vi "Test SyncStart 2.vi"() -> ()   [LabVIEW 2017]
uses:
  274801fc-fe2a-4412-a660-e416e3d3dfa2.vi
  e6d22657-482a-40f8-b9e6-8851e5ea81f9.vi
  9ccd6827-3ff4-4c10-ac1b-fb27d356ceb2.vi
  815a932d-7b12-48c6-9f28-7d788b7c90a6.vi
  25f0e5d1-a262-4e62-8561-2edca888c82f.vi
  Synchronization/SyncStart/_Obtain SyncStart Queue.vi
panel:
  in  "state 3":bool
  in  "state 2":bool
  in  "state 1":bool
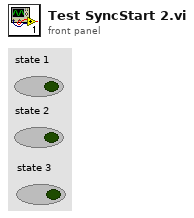
[diagram p1: front panel]
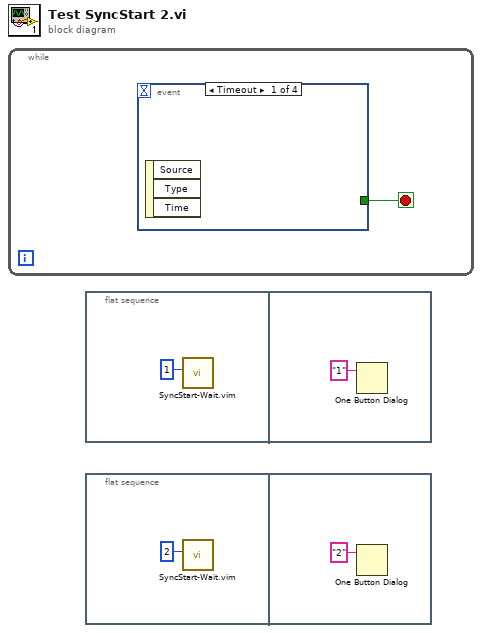
[diagram p0: block diagram]
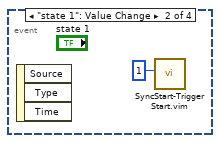
[diagram p2: hidden frame]
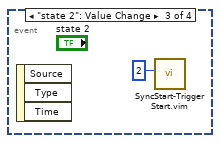
[diagram p3: hidden frame]
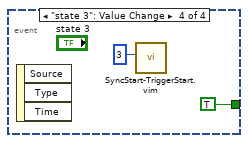
[diagram p4: hidden frame]
diagram:
  n1 = while {
    stop <- w1 stop-if-true
    n2 = event shown="[0] Timeout" {
      selector: _ -> [_ _ _ _]
      dyn-events: _ -> [_ _ _ _]
      timeout: _ -> [_ _ _ _]
      tunnel: [_ _ _ TRUE] -> w1
      event Timeout {
        n3 = event-data() -> ()  [unwired: 1 in, 3 out]
      }
      event "state 1": Value Change {
        n4 = event-data() -> ()  [unwired: 1 in, 3 out]
        n5 = call "SyncStart-TriggerStart.vim"("state(Enum or Int)"=1 ("state")) -> ()  [unwired: 10 in, 1 out]
      }
      event "state 2": Value Change {
        n6 = event-data() -> ()  [unwired: 1 in, 3 out]
        n7 = call "SyncStart-TriggerStart.vim"("state(Enum or Int)"=2 ("state")) -> ()  [unwired: 10 in, 1 out]
      }
      event "state 3": Value Change {
        n8 = event-data() -> ()  [unwired: 1 in, 3 out]
        n9 = call "SyncStart-TriggerStart.vim"("state(Enum or Int)"=3 ("state")) -> ()  [unwired: 10 in, 1 out]
      }
    }
  }
  n10 = flat-sequence {
    frame #0 {
      n11 = call "SyncStart-Wait.vim"("state(Enum or Int)"=1 ("state")) -> ()  [unwired: 10 in, 1 out]
    }
    frame #1 {
      n12 = One Button Dialog(message="1") -> ()  [unwired: 1 in, 1 out]
    }
  }
  n13 = flat-sequence {
    frame #0 {
      n14 = call "SyncStart-Wait.vim"("state(Enum or Int)"=2 ("state")) -> ()  [unwired: 10 in, 1 out]
    }
    frame #1 {
      n15 = One Button Dialog(message="2") -> ()  [unwired: 1 in, 1 out]
    }
  }
